vi "SonarK.vi"(11 "FPGA I/O In":refnum<k21>="Port0/DIO6") -> (1 "Error in System":bool, 2 "Timed Out":bool, 3 "Output":i32)   [LabVIEW 2013]
uses:
  <vilib>/Platform/TimedLoop/XDataNode/timing_clust.ctl
  <vilib>/Platform/TimedLoop/XDataNode/nitl_modes.ctl
  <vilib>/Platform/TimedLoop/XDataNode/wakeup.ctl
  <vilib>/rvi/eio/common/nirviEmuTemplateMethod_errors.vi
  <vilib>/rvi/Emulation/niFpgaSctlEmulationGetInTimedLoop.vi
  <vilib>/rvi/Emulation/niFpgaEmulationReportErrorSimple.vi
  <vilib>/rvi/Emulation/niFpgaGetClockAttributes.vi
  <vilib>/rvi/Emulation/niFpgaCriticalErrorInLSC.vi
  <vilib>/eio/EIOMethodNode/EIOMethodNode.xnode
  <vilib>/eio/EIONode/EIONode.xnode
  <vilib>/Platform/TimedLoop/XDataNode/XDataNode.xnode
  <vilib>/Platform/TimedLoop/XDataNode/XDNodeRunTimeDep.lvlib
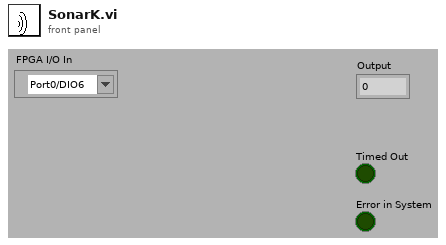
[diagram p1: front panel]
types:
  T1 = typedef "XDNodeRunTimeDep.lvlib/timing_clust.ctl" = cluster{"Expected End [f-1]":u64, "Actual End [f-1]":u64, "Finished Late? [f-1]":bool, "Expected End [i-1]":u64, "Actual End [i-1]":u64, "Finished Late? [i-1]":bool, "Expected Start [i]":u64, "Actual Start [i]":u64, "Expected Start [f]":u64, "Actual Start [f]":u64, "Source Name":string, "Structure Name":string, "Period":i64, "Deadline":i64, "Offset":i64, "Start":i64, "Priority":i32, "Timeout":i32, "Mode":T2, "Wakeup Reason":T3, "Error":errorcluster, "Source Type":string, "Secondary Source Type":string, "Global End Time":u64, "Global Start Time":u64, "Frame Duration":u64, "Iteration Duration":u64, "Assigned CPU":i32, "I/O Scan Engine Mode":u32}
  T2 = typedef "XDNodeRunTimeDep.lvlib/nitl_modes.ctl" = enum32{"No Change", "Process missed periods, maintain original phase", "Discard missed periods, maintain original phase", "Process missed periods, ignore original phase", "Discard missed periods, ignore original phase"}
  T3 = typedef "XDNodeRunTimeDep.lvlib/wakeup.ctl" = enum32{"Normal", "Aborted", "Asynchronous wakeup", "Timing source error", "Timed loop error", "Timeout"}
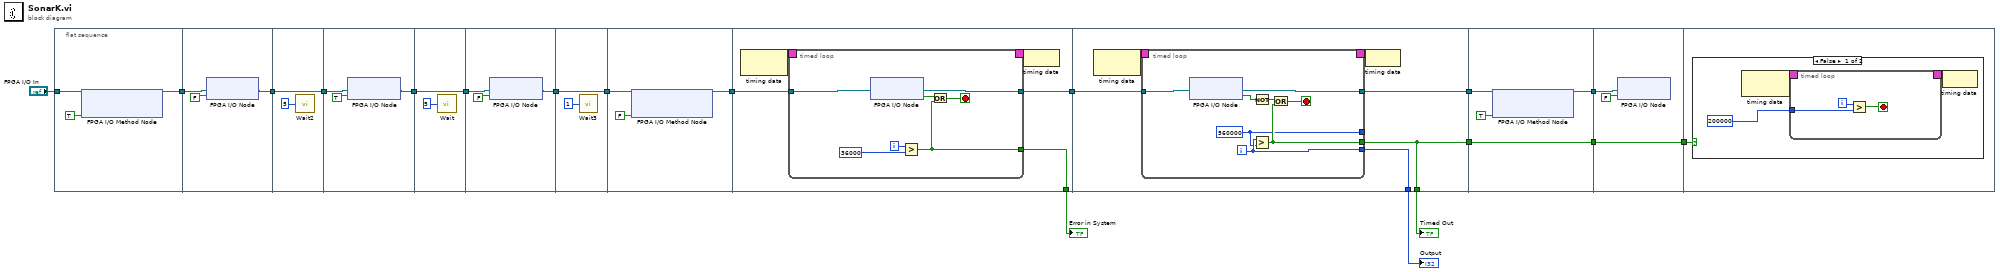
[diagram p0: block diagram]
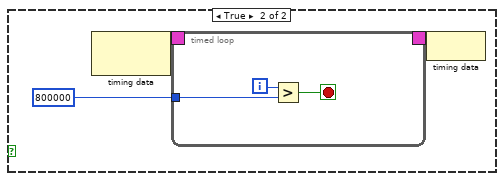
[diagram p2: hidden frame]
diagram:
  n1 = flat-sequence {
    tunnel: "FPGA I/O In" -> [w20]
    tunnel: [w19] -> w13
    tunnel: w13 -> [w23]
    tunnel: [w22] -> w12
    tunnel: w12 -> [w26]
    tunnel: [w26] -> w11
    tunnel: w11 -> [w29]
    tunnel: [w27] -> w17
    tunnel: [w30] -> w10
    tunnel: w17 -> [w30]
    tunnel: w10 -> [w34]
    tunnel: [w33] -> w9
    tunnel: w9 -> [w36]
    tunnel: [w36] -> w8
    tunnel: [w38] -> w16
    tunnel: w8 -> [w37]
    tunnel: w16 -> [w42]
    tunnel: [w41] -> w15
    tunnel: [w40] -> w14
    tunnel: w15 -> [w59]
    tunnel: [w58] -> w7
    tunnel: [w56] -> w4
    tunnel: [w57] -> w6
    tunnel: [w56] -> w1
    tunnel: w7 -> [w76]
    tunnel: [w75] -> w5
    tunnel: [w74] -> w2
    tunnel: w1 -> [w74]
    tunnel: w5 -> [w80]
    tunnel: [w78] -> w3
    tunnel: w2 -> [w78]
    tunnel: w3 -> [w81]
    frame #0 {
      n2 = xnode "FPGA I/O Method Node"("FPGA I/O In"=w20, "Enable"=TRUE) -> ("FPGA I/O Out"=w19:refnum<k21>)
    }
    frame #1 {
      n3 = xnode "FPGA I/O Node"("I/O Item"=FALSE, "FPGA I/O In"=w23) -> ("FPGA I/O Out"=w22:refnum<k21>)
    }
    frame #2 {
      n4 = call "Wait2"("Count(uSec)"=u8 5) -> ()  [unwired: 1 out]
    }
    frame #3 {
      n5 = xnode "FPGA I/O Node"("I/O Item"=TRUE, "FPGA I/O In"=w29) -> ("FPGA I/O Out"=w27:refnum<k21>)
    }
    frame #4 {
      n6 = call "Wait"("Count(uSec)"=u8 5) -> ()  [unwired: 1 out]
    }
    frame #5 {
      n7 = xnode "FPGA I/O Node"("I/O Item"=FALSE, "FPGA I/O In"=w34) -> ("FPGA I/O Out"=w33:refnum<k21>)
    }
    frame #6 {
      n8 = call "Wait3"("Count(uSec)"=u8 1) -> ()  [unwired: 1 out]
    }
    frame #7 {
      n9 = xnode "FPGA I/O Method Node"("FPGA I/O In"=w37, "Enable"=FALSE) -> ("FPGA I/O Out"=w38:refnum<k21>)
    }
    frame #8 {
      n10 = node-c288() -> (w44:T1)  [unwired: 1 in]
      n11 = timed-loop {
        timing: w44 -> [_]
        timing-out: [_] -> w43
        tunnel: w42 -> [w51]
        tunnel: [w46] -> w41
        tunnel: [w45] -> w40
        i -> [w49]
        stop <- w47 stop-if-true
        n12 = xnode "FPGA I/O Node"("FPGA I/O In"=w51) -> ("I/O Item"=w48:bool, "FPGA I/O Out"=w46:refnum<k21>)
        n13 = Greater?(x=w49, y=36000) -> (0:w45:bool)
        n14 = Or(x=w48, y=w45) -> (x .or. y?=w47:bool)
      }
      n15 = node-c288(w43) -> ()
    }
    frame #9 {
      n16 = node-c288() -> (w61:T1)  [unwired: 1 in]
      n17 = timed-loop {
        timing: w61 -> [_]
        timing-out: [_] -> w60
        tunnel: w59 -> [w69]
        tunnel: [w65] -> w57
        tunnel: [w64] -> w56
        tunnel: [w63] -> w58
        tunnel: [w62] -> _
        i -> [w65]
        stop <- w66 stop-if-true
        w62 = 560000
        n18 = xnode "FPGA I/O Node"("FPGA I/O In"=w69) -> ("I/O Item"=w68:bool, "FPGA I/O Out"=w63:refnum<k21>)
        n19 = Not(x=w68) -> (.not. x?=w67:bool)
        n20 = Greater?(x=w65, y=w62) -> (0:w64:bool)
        n21 = Or(x=w67, y=w64) -> (x .or. y?=w66:bool)
      }
      n22 = node-c288(w60) -> ()
    }
    frame #10 {
      n23 = xnode "FPGA I/O Method Node"("FPGA I/O In"=w76, "Enable"=TRUE) -> ("FPGA I/O Out"=w75:refnum<k21>)
    }
    frame #11 {
      n24 = xnode "FPGA I/O Node"("I/O Item"=FALSE, "FPGA I/O In"=w80) -> ()  [unwired: 1 out]
    }
    frame #12 {
      n25 = case shown="False" w81 {
        frame False {
          n26 = node-c288() -> (w84:T1)  [unwired: 1 in]
          n27 = timed-loop {
            timing: w84 -> [_]
            timing-out: [_] -> w83
            tunnel: 200000 ("Wait Count") -> [w86]
            i -> [w87]
            stop <- w85 stop-if-true
            n28 = Greater?(x=w87, y=w86) -> (0:w85:bool)
          }
          n29 = node-c288(w83) -> ()
        }
        frame True {
          n30 = node-c288() -> (w94:T1)  [unwired: 1 in]
          n31 = timed-loop {
            timing: w94 -> [_]
            timing-out: [_] -> w93
            tunnel: 800000 -> [w96]
            i -> [w97]
            stop <- w95 stop-if-true
            n32 = Greater?(x=w97, y=w96) -> (0:w95:bool)
          }
          n33 = node-c288(w93) -> ()
        }
      }
    }
  }
  "Output" <- w6
  "Error in System" <- w14
  "Timed Out" <- w4
